vi "test_sweep.vi"() -> ()   [LabVIEW 2024]
uses:
  AD2_WFG_SDK_class/WFG.ctl
  AD2_WFG_SDK_class/WFGCh.ctl
  AD2_WFG_SDK_class/AD2TriggerSources.ctl
  AD2_MSO_SDK_class/MSOConfig.ctl
  AD2_MSO_SDK_class/AD2TriggerSources.ctl
  AD2_MSO_SDK_class/MSORangeCh.ctl
  AD2_SDK_class/AD2_SDK.lvclass
  <vilib>/Analysis/NI_AALPro.lvlib
  AD2_WFG_SDK_class/AD2_WFG_SDK.lvclass
  AD2_MSO_SDK_class/AD2_MSO_SDK.lvclass
panel:
  out "Power Spectrum":cluster{"Power Spectrum (V^2 rms)":dbl[], dbl[]}(graph)
  in  "Config":T1={"Timing"={"Enable"=TRUE, "Samples In"=0.0, "Sample Rate"=0.0, "Mode"=enum."Single Sample"}, "Trigger"={"Hysteresis"=0.0, "Trigger Level"=0.0, "Trigger Condition"=0, "Trigger Type"=0, "Trigger Channel"=0, "secTimeout"=0.0, "TrigrSrc"=enum."trigrsrcNone"}, "Range Ch1"={"idxChannel"=0, "voltOffset"=0.0, "VoltsRange"=0}, "Range Ch 2"={"idxChannel"=0, "voltOffset"=0.0, "VoltsRange"=0}} {"Range Ch 2"."VoltsRange" items=["High 50V"=50, "Low5V"=5]; "Range Ch1"."VoltsRange" items=["High 50V"=50, "Low5V"=5]; "Trigger"."Trigger Channel" items=["Channel 1"=0, "Channel 2"=1, "Both"=-1]; "Trigger"."Trigger Type" items=["Edge", "Pulse", "Transition"]; "Trigger"."Trigger Condition" items=["Rising", "Falling"]}
  out "Waveform Graph":waveform(dbl)[](graph)
  in  "Freq Sweep (Ch1)":T4
  in  "WFGConfig":T5={"Running"=FALSE, "Ch1"={"idxChannel"=0, "Settings out of range"=FALSE, "Carrier"={"Frequency (Hz)"=0.0, "Amplitude (V)"=1.0, "Offset(V)"=0.0, "Symmetry(%) "=50.0, "Phase(Deg)"=0.0, "Function"=0, "Enable"=FALSE}, "Trigger"={"secRun(0=Cont)"=0.0, "secWait"=0.0, "cRepeat(0=inf)"=0, "Repeat Trigger"=FALSE, "TrigrSrc"=enum."trigrsrcNone"}, "FM Mod"={"Frequency (Hz)"=1000.0, "Amplitude (%)"=1.0, "Offset(V)"=0.0, "Symmetry(%) "=50.0, "Phase(Deg)"=0.0, "Function 2"=1, "Enable"=FALSE}}, "Ch2"={"idxChannel"=1, "Settings out of range"=FALSE, "Carrier"={"Frequency (Hz)"=1000.0, "Amplitude (V)"=1.0, "Offset(V)"=0.0, "Symmetry(%) "=50.0, "Phase(Deg)"=0.0, "Function"=1, "Enable"=FALSE}, "Trigger"={"secRun(0=Cont)"=0.0, "secWait"=0.0, "cRepeat(0=inf)"=0, "Repeat Trigger"=FALSE, "TrigrSrc"=enum."trigrsrcNone"}, "FM Mod"={"Frequency (Hz)"=1000.0, "Amplitude (%)"=1.0, "Offset(V)"=0.0, "Symmetry(%) "=50.0, "Phase(Deg)"=0.0, "Function 2"=1, "Enable"=FALSE}}, "SyncronizeState"=enum."Independent"} {"Ch2"."FM Mod"."Function 2" items=["DC"=0, "Sine"=1, "Square"=2, "Triangle"=3, "RampUp"=4, "RampDown"=5, "Noise"=6, "Pulse"=7, "Custom"=30]; "Ch2"."Carrier"."Function" items=["DC"=0, "Sine"=1, "Square"=2, "Triangle"=3, "RampUp"=4, "RampDown"=5, "Noise"=6, "Pulse"=7, "Custom"=30]; "Ch1"."FM Mod"."Function 2" items=["DC"=0, "Sine"=1, "Square"=2, "Triangle"=3, "RampUp"=4, "RampDown"=5, "Noise"=6, "Pulse"=7, "Custom"=30]; "Ch1"."Carrier"."Function" items=["DC"=0, "Sine"=1, "Square"=2, "Triangle"=3, "RampUp"=4, "RampDown"=5, "Noise"=6, "Pulse"=7, "Custom"=30]}
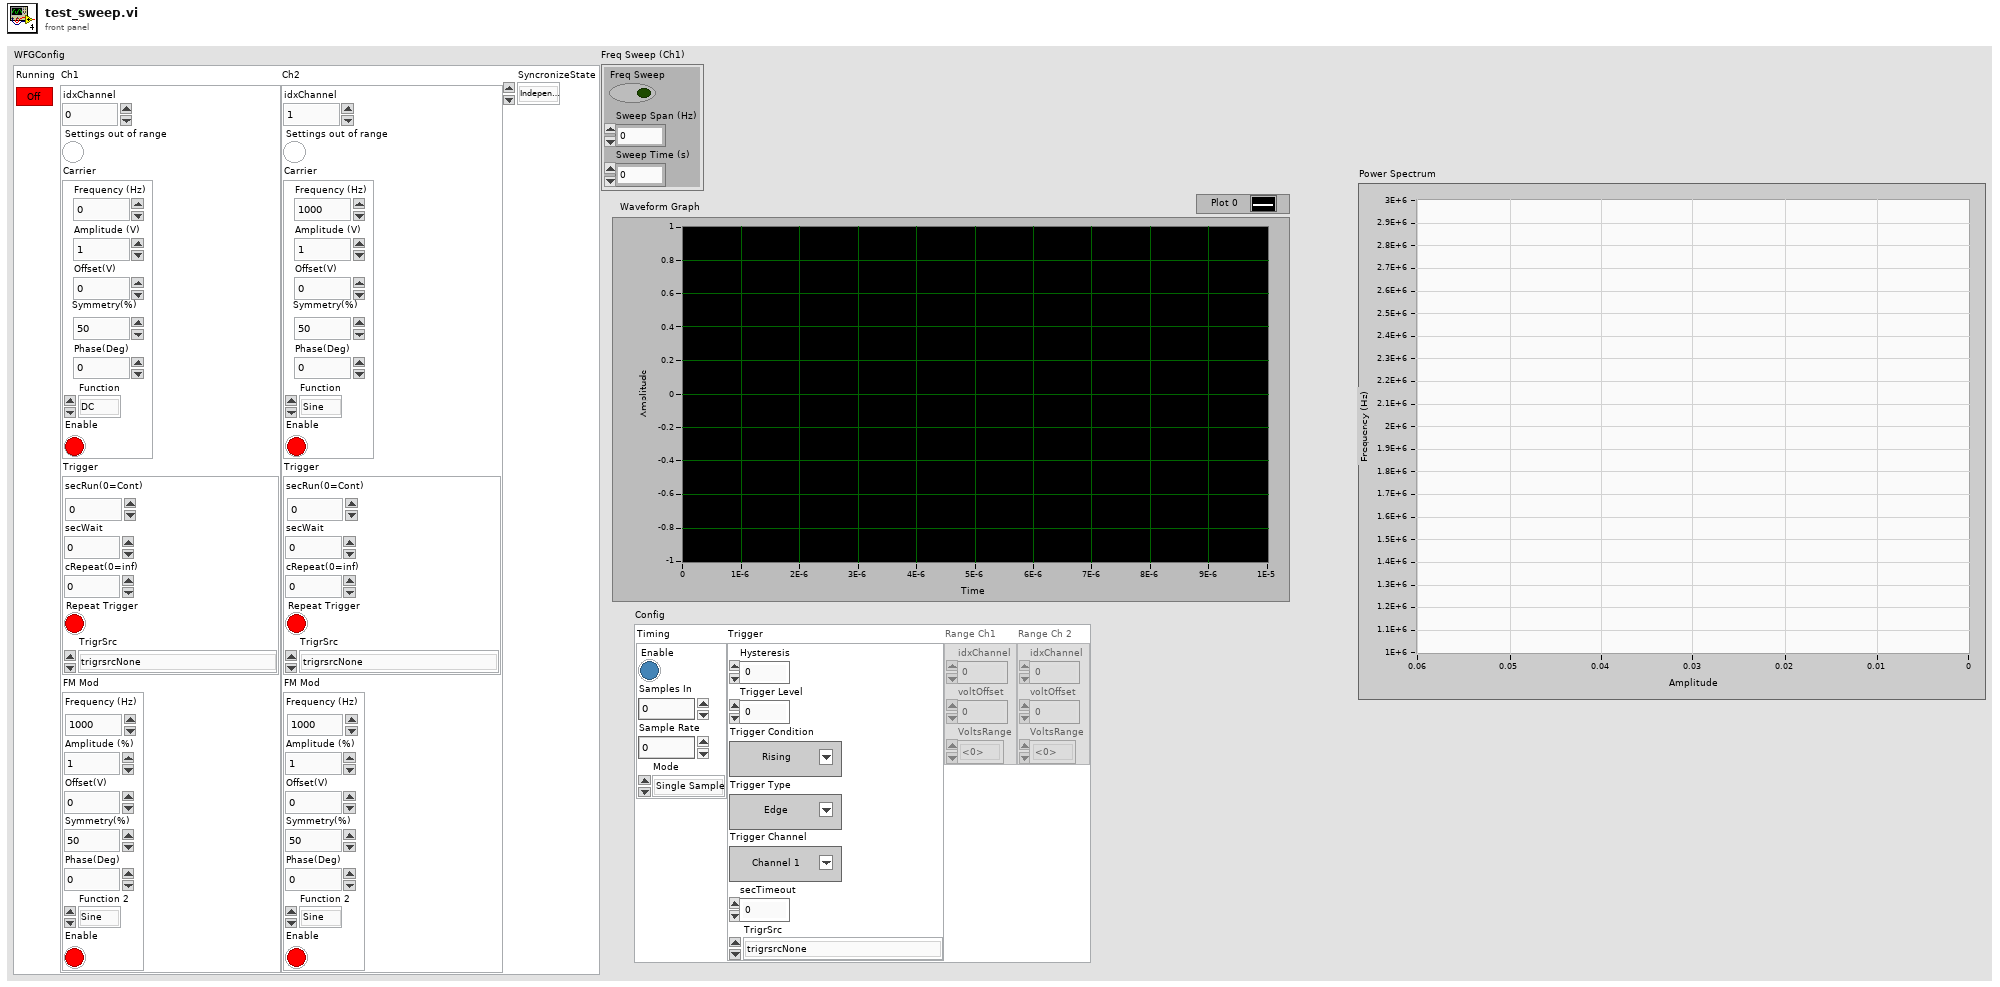
[diagram p1: front panel]
types:
  T1 = typedef "AD2_MSO_SDK.lvclass/MSOConfig.ctl" = cluster{"Timing":cluster{"Enable":bool, "Samples In":dbl, "Sample Rate":dbl, "Mode":enum16{"Single Sample", "Scanshift", "Multiple Samples", "Scan Screen"}}, "Trigger":cluster{"Hysteresis":dbl, "Trigger Level":dbl, "Trigger Condition":i32, "Trigger Type":i32, "Trigger Channel":i32, "secTimeout":dbl, "TrigrSrc":T2}, "Range Ch1":T3, "Range Ch 2":T3}
  T2 = typedef "AD2_MSO_SDK.lvclass/AD2TriggerSources.ctl" = enum8{"trigrsrcNone", "trigsrcPC", "trigsrcDetectorAnalogIn", "trigsrcDetectorDigitalIn", "trigsrcAnalogIn", "trigsrcDigitalIn", "trigsrcDigitalOut", "trigsrcAnalogOut1", "trigsrcAnalogOut2", "trigsrcAnalogOut3", "trigsrcAnalogOut4", "trigsrcExternal1", "trigsrcExternal2", "trigsrcExternal3", "trigsrcExternal4", ""}
  T3 = typedef "AD2_MSO_SDK.lvclass/MSORangeCh.ctl" = cluster{"idxChannel":i32, "voltOffset":dbl, "VoltsRange":u16}
  T4 = cluster{"Freq Sweep":bool, "Sweep Span (Hz)":dbl, "Sweep Time (s)":dbl}
  T5 = typedef "AD2_WFG_SDK.lvclass/WFG.ctl" = cluster{"Running":bool, "Ch1":T6, "Ch2":T6, "SyncronizeState":enum16{"Independent", "Ch1Master", "Ch2Master"}}
  T6 = typedef "AD2_WFG_SDK.lvclass/WFGCh.ctl" = cluster{"idxChannel":i32, "Settings out of range":bool, "Carrier":cluster{"Frequency (Hz)":dbl, "Amplitude (V)":dbl, "Offset(V)":dbl, "Symmetry(%) ":dbl, "Phase(Deg)":dbl, "Function":u16, "Enable":bool}, "Trigger":cluster{"secRun(0=Cont)":dbl, "secWait":dbl, "cRepeat(0=inf)":i32, "Repeat Trigger":bool, "TrigrSrc":T7}, "FM Mod":cluster{"Frequency (Hz)":dbl, "Amplitude (%)":dbl, "Offset(V)":dbl, "Symmetry(%) ":dbl, "Phase(Deg)":dbl, "Function 2":u16, "Enable":bool}}
  T7 = typedef "AD2_SDK.lvclass/AD2TriggerSources.ctl" = enum8{"trigrsrcNone", "trigsrcPC", "trigsrcDetectorAnalogIn", "trigsrcDetectorDigitalIn", "trigsrcAnalogIn", "trigsrcDigitalIn", "trigsrcDigitalOut", "trigsrcAnalogOut1", "trigsrcAnalogOut2", "trigsrcAnalogOut3", "trigsrcAnalogOut4", "trigsrcExternal1", "trigsrcExternal2", "trigsrcExternal3", "trigsrcExternal4", ""}
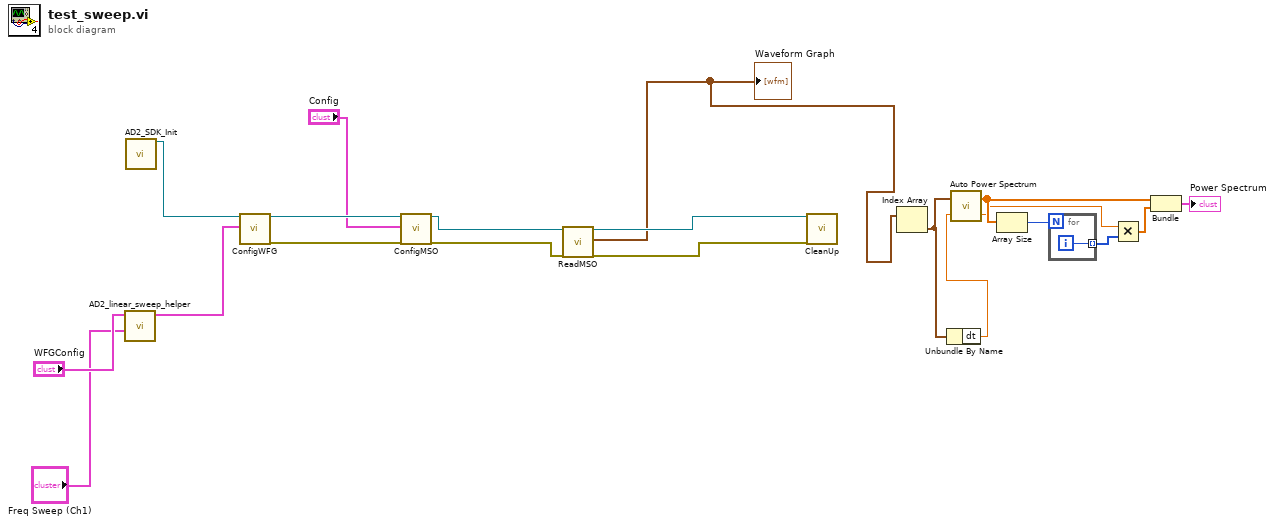
[diagram p0: block diagram]
diagram:
  n1 = call "AD2_linear_sweep_helper.vi"("Freq Sweep (Ch1)"="Freq Sweep (Ch1)", "WFGConfig"="WFGConfig") -> ("WFGConfig 2"=w19:T5)  [unwired: 9 in]
  n2 = call "AD2_SDK_Init.vi"() -> ("object out"=w17:refnum<class "AD2_SDK.lvclass">)  [unwired: 18 in, 1 out]
  n3 = call-dynamic "ConfigWFG.vi"("object in"=w17, "Config(var)"=w19) -> ("object out"=w16:refnum<class "AD2_SDK.lvclass">, "error out"=w15:errorcluster)  [unwired: 16 in]
  n4 = call-dynamic "ConfigMSO.vi"("object in"=w16, "variant"="Config", "error in (no error)"=w15) -> ("object out"=w14:refnum<class "AD2_SDK.lvclass">, "error out"=w13:errorcluster)  [unwired: 15 in]
  n5 = call-dynamic "ReadMSO.vi"("object in"=w14, "error in (no error)"=w13) -> ("object out"=w12:refnum<class "AD2_SDK.lvclass">, "Channels array"=w3:waveform(dbl)[], "error out"=w11:errorcluster)  [unwired: 15 in]
  "Waveform Graph" <- w3
  n6 = call-dynamic "CleanUp.vi"("object in"=w12, "error in (no error)"=w11) -> ()  [unwired: 16 in, 2 out]
  n7 = Index Array(array=w3) -> (element=w1:waveform(dbl))  [unwired: 1 in]
  n8 = Unbundle By Name(w1) -> ("dt"=w2:dbl)
  n9 = call <vilib>:"Auto Power Spectrum.vi"("dt"=w2, "Signal (V)"=w1) -> ("df"=w6:dbl, "Power Spectrum (V^2 rms)"=w7:dbl[])
  n10 = Array Size(array=w7) -> (size(s)=w8:i32)
  n11 = for {
    N: w8 -> [_]
    tunnel: [w21] -> w5 mode=indexing
    i -> [w21]
  }
  n12 = Multiply(x=w6, y=w5) -> (x*y=w4:dbl[])
  n13 = Bundle("Power Spectrum (V^2 rms)"=w7, w4) -> (→"Power Spectrum":cluster{"Power Spectrum (V^2 rms)":dbl[], dbl[]})  [unwired: 1 out]
